vi "Save_stimuli.vi"(0 "Array":T1(array[cluster])) -> ()   [LabVIEW 2016]
uses:
  <vilib>/Utility/xml.llb/Write to XML File(string).vi
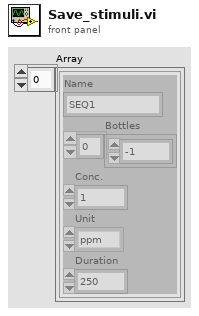
[diagram p1: front panel]
types:
  T1 = cluster{"Name":string, "Bottles":i32[], "Conc.":dbl, "Unit":enum16{"%", "ppm"}, "Duration":dbl}[]
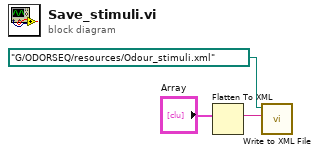
[diagram p0: block diagram]
diagram:
  n1 = Flatten To XML(anything="Array") -> (xml string=w2:string)
  n2 = call-poly <vilib>:"Write to XML File.vi"("XML Input"=w2, "XML File Path"=path "G:/ODORSEQ/resources/Odour_stimuli.xml") -> ()  [unwired: 7 in, 3 out]
